vi "Get Record Count.vi"(9 "Offset in":i32, 10 "Bytes in":u8[](array[numeric]) format="%.0x", 11 "pcap_Parse_Build_CIF":refnum<class "pcap_Parse_Build_CIF.lvclass">) -> (2 "Records":i32)   [LabVIEW 2021, in "pcap_Parse_Build_CIF.lvclass"]
uses:
  pcap_Parse_Build_CIF.lvclass
  pcap_Parse_Build_CIF.lvclass/pcap_Parse_Build_CIF.ctl
  <vilib>/CIF Foundation/CIF Utilities/DataTypes/DataTypes_CIF_U.lvlib
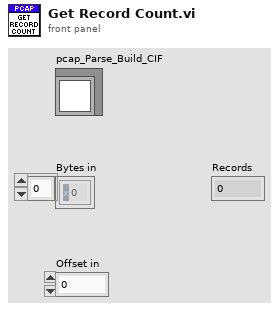
[diagram p1: front panel]
types:
  T1 = typedef "DataTypes_CIF_U.lvlib/Endian.ctl" = enum16{"Little Endian", "Big Endian"}
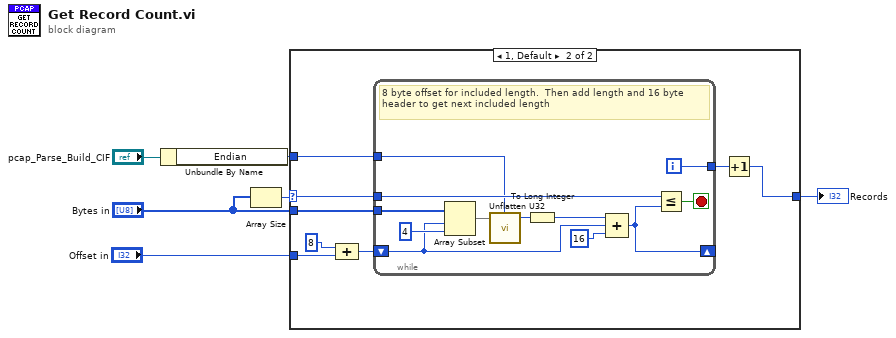
[diagram p0: block diagram]
diagram:
  n1 = Unbundle By Name("pcap_Parse_Build_CIF") -> ("Endian"=w3:T1)
  n2 = Array Size(array="Bytes in") -> (size(s)=w2:i32)
  n3 = case shown="1, Default" w2 {
    selector: w2 -> [w7 w11]
    tunnel: "Bytes in" -> [_ w15]
    tunnel: [w7 w14] -> w4
    tunnel: w3 -> [_ w13]
    tunnel: "Offset in" -> [_ w10]
    frame 0 {
    }
    frame 1, Default {
      n4 = Compound Arithmetic op=ADD(8 ("Offset"), w10) -> (w9:i32)
      n5 = while {
        tunnel: w11 -> [w26]
        tunnel: [w25] -> w12
        tunnel: w15 -> [w22]
        shift-right: [w21] -> _
        shift-left: w9 -> [w18]
        tunnel: w13 -> [w16]
        i -> [w25]
        stop <- w27 stop-if-true
        # "8 byte offset for included length.  Then add length and 16 byte header to get next included length"
        n6 = Array Subset(array=w22, index=w18, length=4 ("index")) -> (w23:u8[])
        n7 = call <vilib>:"Unflatten U32.vi"("Flat Data"=w23, "Endian"=w16) -> ("U32"=w20:u32)  [unwired: 3 in]
        n8 = To Long Integer(number=w20) -> (32bit integer=w19:i32)
        n9 = Compound Arithmetic op=ADD(w19, w18, 16 ("value")) -> (w21:i32)
        n10 = Less Or Equal?(x=w26, y=w21) -> (x <= y?=w27:bool)
      }
      n11 = Increment(x=w12) -> (x+1=w14:i32)
    }
  }
  "Records" <- w4
